vi "Configure Power Factor.vi"(8 "error in (no error)":errorcluster, 9 "Phase Offset Type (0: Lead)":i32(ring) items=["Lead", "Lag"], 10 "Power Factor (1.0)":dbl=1.0, 11 "VISA resource name":refnum<visa-resource-name>) -> (0 "error out":errorcluster, 3 "VISA resource name out":refnum<visa-resource-name>)   [LabVIEW 2012, in "Fluke 5080.lvlib"]
doc: "Sets the displacement power factor (phase angle) between the NORMAL and AUX terminals."
uses:
  <instrlib>/Fluke 5080/Fluke 5080.lvlib
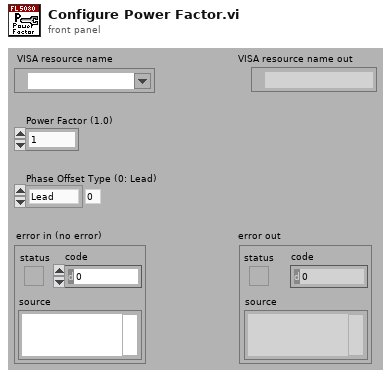
[diagram p1: front panel]
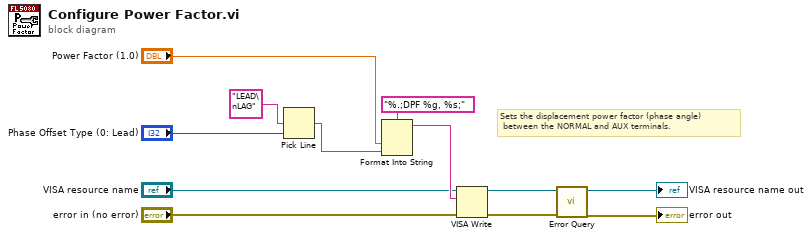
[diagram p0: block diagram]
diagram:
  # "Sets the displacement power factor (phase angle)\n between the NORMAL and AUX terminals."
  n1 = Pick Line(multi-line string="LEAD\nLAG", line index="Phase Offset Type (0: Lead)") -> (output string=w8:string)  [unwired: 1 out]
  n2 = Format Into String(format string="%.;DPF %g, %s;", "Power Factor (1.0)", w8) -> (resulting string=w7:string)  [unwired: 2 in, 1 out]
  n3 = VISA Write(VISA resource name="VISA resource name", write buffer=w7, error in (no error)="error in (no error)") -> (VISA resource name out=w4:refnum<visa-resource-name>, error out=w3:errorcluster)  [unwired: 1 out]
  n4 = call <instrlib>:"Error Query.vi"("error in (no error)"=w3, "VISA resource name"=w4) -> ("error out"=→"error out":errorcluster, "VISA resource name out"=→"VISA resource name out":refnum<visa-resource-name>)  [unwired: 8 out]
